vi "Write Data.vi"(8 "error in (no error)":errorcluster, 9 "Publication Time":timestamp, 10 "Value":variant, 11 "MCListboxItemNamesBinding In":refnum<class "MCListboxItemNamesBinding.lvclass">) -> (0 "error out":errorcluster, 3 "MCListboxItemNamesBinding Out":refnum<class "MCListboxItemNamesBinding.lvclass">)   [LabVIEW 2015, in "Transport.lvlib" / "MCListboxItemNamesBinding.lvclass"]
doc: "<License>\nCopyright © 2017 Composed Systems, LLC | All rights reserved\nwww.composed.io\n\nAuthor: Ethan Stern <ethan.stern@composed.io>\n\nThis software is provided \"AS IS\" WITHOUT WARRANTIES, either express or implied, AND IS FOR EDUCATIONAL PURPOSES ONLY.\n</License>"
uses:
  MCListboxItemNamesBinding.lvclass
  MCListboxItemNamesBinding.lvclass/MCListboxItemNamesBinding.ctl
  <vilib>/Utility/error.llb/Error Cluster From Error Code.vi
  <vilib>/ErrorRing/Error Ring.xnode
  <vilib>/Utility/Data Type/NI_Data Type.lvlib
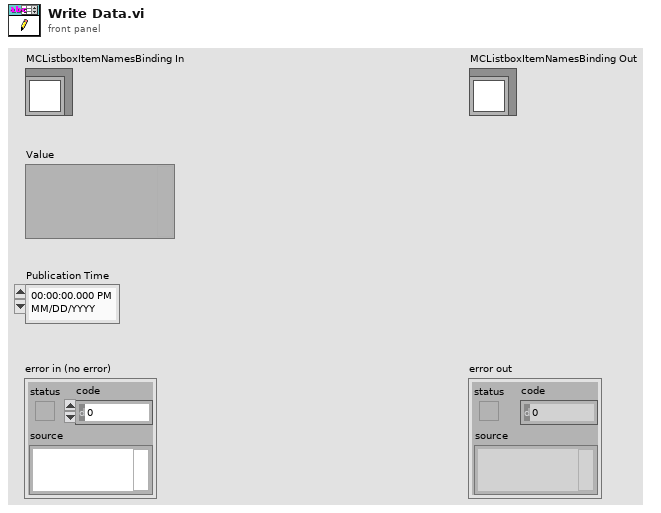
[diagram p1: front panel]
types:
  T1 = typedef "NI_Data Type.lvlib/Data Type.ctl" = enum8{"Invalid Type", "Void", "I8", "I16", "I32", "I64", "U8", "U16", "U32", "U64", "Single Float", "Double Float", "Extended Float", "Single Complex", "Double Complex", "Extended Complex", "Enum U8", "Enum U16", "Enum U32", "Enum U64", "Single Float With Unit", "Double Float With Unit", "Extended Float With Unit", "Single Complex with Unit", "Double Complex with Unit", "Extended Complex with Unit", "Boolean", "String", "Path", "Picture", "Tag", "Array", "Cluster", "Variant", "LV Variant", "Waveform", "Timestamp", "Digital Waveform", "Digital Data", "ExpressData", "Refnum", "External Data", "VI", "Poly VI", "LabVIEW Class Instance", "Fixed Point"}
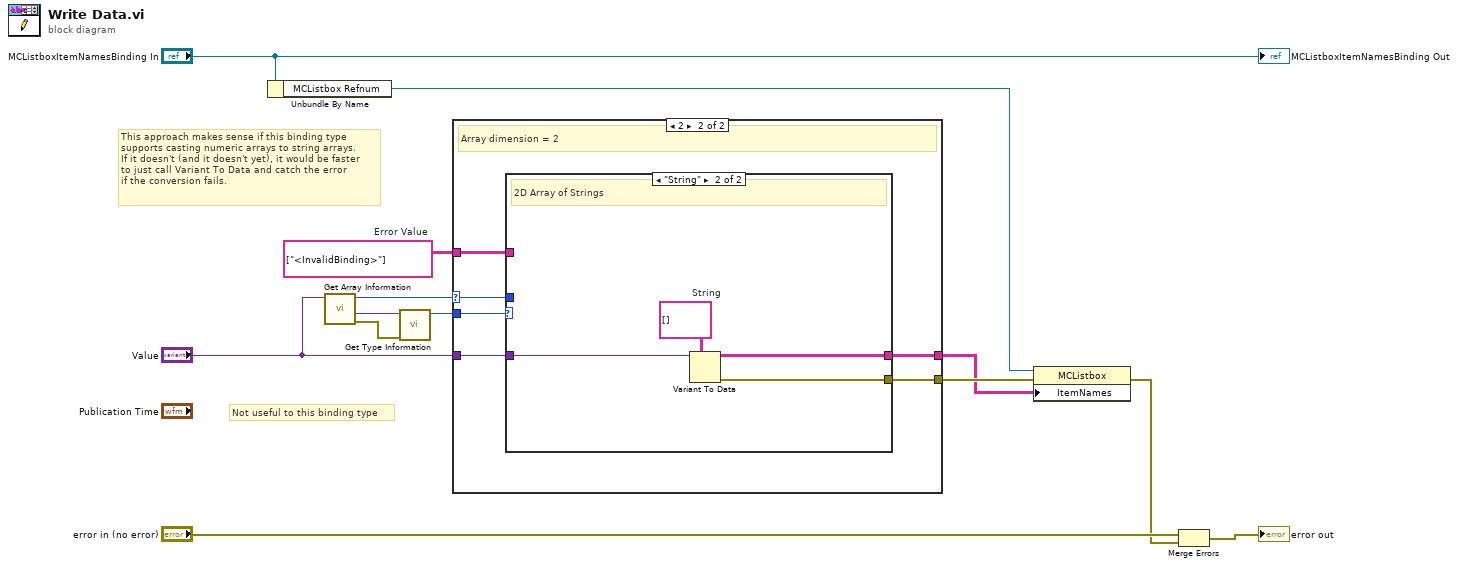
[diagram p0: block diagram]
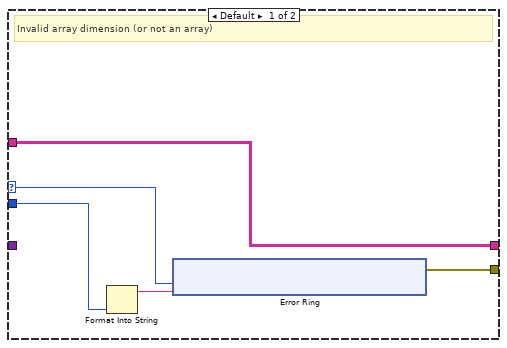
[diagram p2: hidden frame]
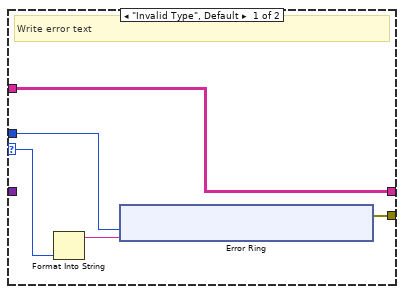
[diagram p3: hidden frame]
diagram:
  w2 = string[][] [["<InvalidBinding>"]]  # Error Value
  # "This approach makes sense if this binding type\nsupports casting numeric arrays to string arrays.\nIf it doesn't (and it doesn't yet), it would be faster\nto just call Variant To Data and catch the error\nif the conversion fails."
  # "Not useful to this binding type"
  n1 = Unbundle By Name("MCListboxItemNamesBinding In") -> ("MCListbox Refnum"=w10:refnum<vi>)
  n2 = call <vilib>:"Get Array Information.vi"("Variant"="Value") -> ("error out"=w1:errorcluster, "Array Element Data Type"=w6:variant, "Number of Dimensions"=w4:i32)  [unwired: 7 in, 1 out]
  n3 = call <vilib>:"Get Type Information.vi"("error in (no error)"=w1, "Variant"=w6) -> ("Type"=w3:T1)  [unwired: 5 in, 4 out]
  n4 = case shown="2" w4 {
    selector: w4 -> [w15 w28]
    tunnel: [w16 w32] -> w8
    tunnel: [w18 w31] -> w7
    tunnel: "Value" -> [_ w30]
    tunnel: w3 -> [w14 w29]
    tunnel: w2 -> [w18 w27]
    frame Default {
      # "Invalid array dimension (or not an array)"
      n5 = Format Into String(w14) -> (resulting string=w17:string)  [unwired: 3 in, 1 out]
      n6 = xnode "Error Ring"("parameter 0"=w15, "parameter 1"=w17) -> ("error out"=w16:errorcluster)
    }
    frame 2 {
      # "Array dimension = 2"
      n7 = case shown="\"String\"" w29 {
        selector: w29 -> [w36 _]
        tunnel: w30 -> [_ w49]
        tunnel: [w37 w46] -> w32
        tunnel: [w33 w47] -> w31
        tunnel: w28 -> [w34 _]
        tunnel: w27 -> [w33 _]
        frame "Invalid Type", Default {
          # "Write error text"
          n8 = Format Into String(w36) -> (resulting string=w35:string)  [unwired: 3 in, 1 out]
          n9 = xnode "Error Ring"("parameter 0"=w34, "parameter 1"=w35) -> ("error out"=w37:errorcluster)
        }
        frame "String" {
          w48 = string[][] []  # String
          # "2D Array of Strings"
          n10 = Variant To Data(type=w48, Variant=w49) -> (data=w47:string[][], error out=w46:errorcluster)  [unwired: 1 in]
        }
      }
    }
  }
  n11 = property class="MCListbox"(reference=w10, error in=w8, "ItemNames"=w7) -> (error out=w9:errorcluster)  [unwired: 1 out]
  n12 = Merge Errors("error in (no error)", w9) -> (→"error out":errorcluster)
  "MCListboxItemNamesBinding Out" <- "MCListboxItemNamesBinding In"
